vi "Target x Location.vi"() -> ()   [LabVIEW 2016]
panel:
  out "Target x Location indic":dbl
  in  "Target x Location contr":dbl
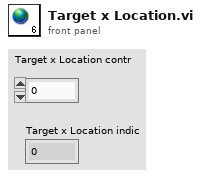
[diagram p1: front panel]
diagram:
